vi "Init.vi"(11 "Game Play Type":refnum<vi>) -> (3 "cluster out":T1)   [LabVIEW 2019]
uses:
  Main VI references.ctl
  main queue data type.ctl
  top level commands.ctl
  error module commands.ctl
  Scene Commands.ctl
  Cube Data Ops.ctl
  Stop Timing Module commands.vi
  Play timing module commands.ctl
panel:
  in  "cluster":T1
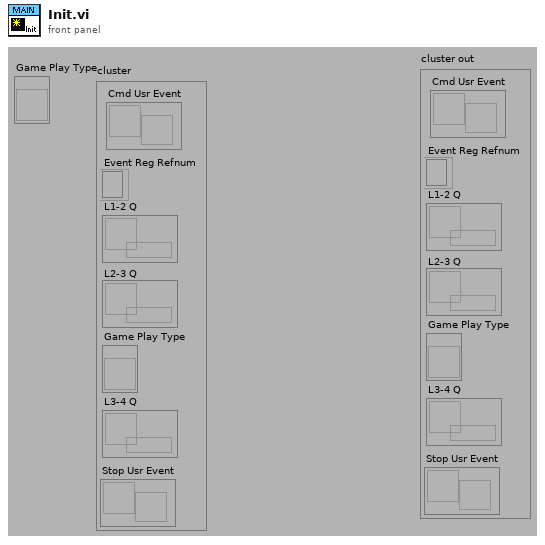
[diagram p1: front panel]
types:
  T1 = typedef "Main VI references.ctl" = cluster{"Cmd Usr Event":refnum<user-event>, "Event Reg Refnum":refnum<event-registration>, "L1-2 Q":refnum<queue>, "L2-3 Q":refnum<queue>, "Game Play Type":refnum<vi>, "L3-4 Q":refnum<queue>, "Stop Usr Event":refnum<user-event>}
  T2 = typedef "error module commands.ctl" = enum16{"Cleanup References", "Set References", "Report Errors", "Process Errors"}
  T3 = typedef "Scene Commands.ctl" = enum16{"Init", "Set Rubix Text Array", "Get Rubix Ref Array", "Generate Rubix Array", "Get Rubix Array", "Show Render Window", "Go To Face", "Rotate", "Update Scene", "Clear Rubix"}
  T4 = typedef "Play timing module commands.ctl" = enum16{"Clean up", "Initialize", "Run"}
  T5 = typedef "Cube Data Ops.ctl" = enum16{"Initialize", "Set Rubix Ref Array", "Set Rubix Text Array", "Set Current Face", "Get Rubix Text Array", "Generate Rubix Array", "Get Rubix array", "Get Facets to move", "Randomize", "Top row left", "Top row right", "Middle row left", "Middle row right", "Bottom row left", "Bottom row right", "Left column up", "Left column down", "Middle column up", "Middle column down", "Right column up", "Right column down", "Face ccw", "Face cw"}
  T6 = typedef "Stop Timing Module commands.vi" = enum16{"Set Name", "Stop loops"}
  T7 = typedef "main queue data type.ctl" = cluster{"Command":T8, "Data":variant}
  T8 = typedef "top level commands.ctl" = enum16{"Idle", "Set Cube Orientation", "Get Cube Orientation", "Go to Face", "Solve", "Test", "Randomize", "Game Play Type", "Stop", "rotate Cube"}
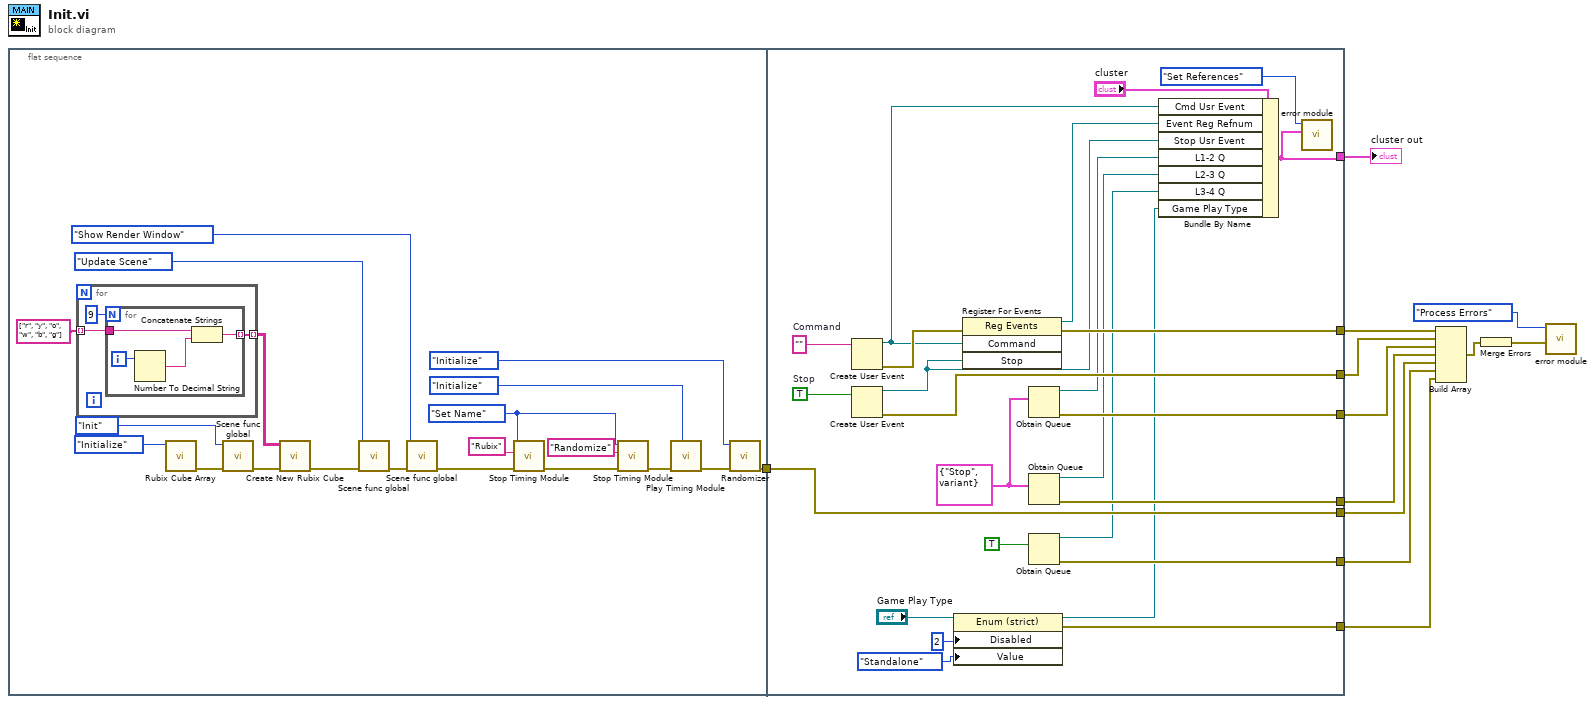
[diagram p0: block diagram]
diagram:
  n1 = flat-sequence {
    tunnel: [w15] -> w6
    tunnel: [w56] -> w12
    tunnel: [w55] -> w10
    tunnel: [w54] -> w9
    tunnel: [w53] -> w8
    tunnel: [w41] -> w1
    tunnel: [w52] -> w11
    tunnel: [w51] -> w5
    tunnel: w6 -> [w51]
    tunnel: [w42] -> w4
    frame #0 {
      w25 = Stop_Timing_Module_commands.vi."Set Name" ("command")
      n2 = for {
        tunnel: string[] ["r", "y", "o", "w", "b", "g"] -> [w35] mode=indexing
        tunnel: [w33] -> w13 mode=indexing
        n3 = for {
          N: 9 -> [_]
          tunnel: w35 -> [w38]
          tunnel: [w36] -> w33 mode=indexing
          i -> [w39]
          n4 = Number To Decimal String(number=w39) -> (decimal integer string=w37:string)  [unwired: 1 in]
          n5 = Concatenate Strings(w38, w37) -> (w36:string)
        }
      }
      n6 = call "Rubix Cube Array.vi"("Command"=Cube_Data_Ops."Initialize") -> ("error out(no error)"=w30:errorcluster)  [unwired: 6 in, 4 out]
      n7 = call "Scene func global.vi"("error in (no error)"=w30, "Commands"=Scene_Commands."Init") -> ("error out"=w21:errorcluster)  [unwired: 8 in, 1 out]
      n8 = call "Create New Rubix Cube.vi"("error out"=w21, "Rubix Array pattern"=w13) -> ("error out(no error)"=w19:errorcluster)  [unwired: 9 in]
      n9 = call "Scene func global.vi"("error in (no error)"=w19, "Commands"=Scene_Commands."Update Scene") -> ("error out"=w17:errorcluster)  [unwired: 8 in, 1 out]
      n10 = call "Scene func global.vi"("error in (no error)"=w17, "Commands"=Scene_Commands."Show Render Window") -> ("error out"=w16:errorcluster)  [unwired: 8 in, 1 out]
      n11 = call "Stop Timing Module.vi"("error in (no error)"=w16, "Structure Names"="Rubix", "command"=w25) -> ("error out"=w27:errorcluster)  [unwired: 8 in]
      n12 = call "Stop Timing Module.vi"("error in (no error)"=w27, "Structure Names"="Randomize", "command"=w25) -> ("error out"=w26:errorcluster)  [unwired: 8 in]
      n13 = call "Play Timing Module.vi"("Commands"=Play_timing_module_commands."Initialize", "error in"=w26) -> ("error out"=w22:errorcluster)  [unwired: 9 in]
      n14 = call "Randomizer.vi"("error in"=w22, "Commands"=Play_timing_module_commands."Initialize") -> ("error out"=w15:errorcluster)  [unwired: 8 in, 1 out]
    }
    frame #1 {
      w64 = ""  # Command
      w63 = TRUE  # Stop
      w61 = T7 {"Command"=enum."Stop", "Data"=variant} ("Cluster")
      n15 = Create User Event(user event datatype=w64) -> (user event=w48:refnum<user-event>, error out=w57:errorcluster)  [unwired: 1 in]
      n16 = Create User Event(user event datatype=w63) -> (user event=w44:refnum<user-event>, error out=w52:errorcluster)  [unwired: 1 in]
      n17 = property class="Enum (strict)"(reference="Game Play Type", "Disabled"=u8 2, "Value"=enum16{"Standalone", "UI Master", "UI Salve"}."Standalone") -> (reference out=w40:refnum<vi>, error out=w41:errorcluster)  [unwired: 1 in]
      n18 = register-events(error in=w57, w48, w44) -> (reference out=w49:refnum<event-registration>, error out=w56:errorcluster)  [unwired: 1 in]
      n19 = Obtain Queue(element data type=w61) -> (queue out=w47:refnum<queue>, error out=w55:errorcluster)  [unwired: 4 in, 1 out]
      n20 = Obtain Queue(element data type=w61) -> (queue out=w46:refnum<queue>, error out=w54:errorcluster)  [unwired: 4 in, 1 out]
      n21 = Obtain Queue(element data type=TRUE) -> (queue out=w45:refnum<queue>, error out=w53:errorcluster)  [unwired: 4 in, 1 out]
      n22 = Bundle By Name(cluster="cluster", "Cmd Usr Event"=w48, "Event Reg Refnum"=w49, "Stop Usr Event"=w44, "L1-2 Q"=w47, "L2-3 Q"=w46, "L3-4 Q"=w45, "Game Play Type"=w40) -> (w42:T1)
      n23 = call "error module.vi"("cluster 2"=w42, "Enum"=error_module_commands."Set References") -> ()  [unwired: 9 in, 1 out]
    }
  }
  n24 = Build Array(w12, w11, w10, w9, w5, w8, w1) -> (w7:errorcluster[])
  n25 = Merge Errors(w7) -> (w3:errorcluster)
  n26 = call "error module.vi"("error in (no error)"=w3, "Enum"=error_module_commands."Process Errors") -> ()  [unwired: 9 in, 1 out]
  "cluster out" <- w4
